vi "Autonomous Independent.vi"   [LabVIEW 2019]
doc: "This VI is called when autonomous begins, and will automatically be terminated when autonomous ends. You can carry out timed or sensor driven robot movement independently without needing to return to the caller."
uses:
  <vilib>/Rock Robotics/WPI/Utilities/WPI_GetSetVariantRefNum.vi
  <vilib>/Rock Robotics/Network Tables/NT Write Numeric Array.vi
  <vilib>/Rock Robotics/Network Tables/NT Read String.vi
panel:
  # "Be sure to right-click and choose Data Operations>>Make Current Value default if you want to save the array values with the VI"
types:
  T1 = typedef "WPI_JoystickDevRef.ctl" = cluster{"Device":T2}
  T2 = typedef "WPI_JoystickDeviceEnum.ctl" = enum16{"USB 0", "USB 1", "USB 2", "USB 3", "USB 4", "USB 5"}
  T3 = typedef "WPI_RobotDriveDevRef.ctl" = cluster{"DevStatus":errorcluster, "Motors[]":T4[], "Square Inputs":bool, "Max Output":dbl}
  T4 = typedef "WPI_MotorControlDeviceRef.ctl" = cluster{"DeviceStatus":errorcluster, "Type":T5, "PWM":cluster{"PWM Channel":T6, "DeadBand":T7}, "CAN":cluster{"Device Number":u8, "SetOutput VI Ref":variant, "GetOutput VI Ref":variant, "Enable VI Ref":variant, "Disable VI Ref":variant, "Data":variant}, "Invert":bool, "DIO PWM":cluster{"PWM \"Enable\" Channel":T6, "DIOChannel":T8, "PWM Rate":dbl}}
  T5 = typedef "WPI_MotorControlType.ctl" = enum16{"PWM", "CAN", "DIO PWM"}
  T6 = typedef "FPGA_DIOPWMChannel.ctl" = enum8{"PWM 0", "PWM 1", "PWM 2", "PWM 3", "PWM 4", "PWM 5", "PWM 6", "PWM 7", "PWM 8", "PWM 9", "PWM MXP 0", "PWM MXP 1", "PWM MXP 2", "PWM MXP 3", "PWM MXP 4", "PWM MXP 5", "PWM MXP 6", "PWM MXP 7", "PWM MXP 8", "PWM MXP 9", "Invalid"}
  T7 = typedef "WPI_PWMDeadband.ctl" = cluster{"Name":string, "maxPositivePwm":i32, "minPositivePwm":i32, "centerPwm":i32, "maxNegativePwm":i32, "minNegativePwm":i32, "angularRange":u16}
  T8 = typedef "FPGA_DIOChannel.ctl" = enum8{"DIO 0", "DIO 1", "DIO 2", "DIO 3", "DIO 4", "DIO 5", "DIO 6", "DIO 7", "DIO 8", "DIO 9", "DIO MXP 0", "DIO MXP 1", "DIO MXP 2", "DIO MXP 3", "DIO MXP 4", "DIO MXP 5", "DIO MXP 6", "DIO MXP 7", "DIO MXP 8", "DIO MXP 9", "DIO MXP 10", "DIO MXP 11", "DIO MXP 12", "DIO MXP 13", "DIO MXP 14", "DIO MXP 15", "SPI Port CS1", "SPI Port CS2", "SPI Port CS3", "SPI Port MISO", "SPI Port MOSI", "Invalid"}
  T9 = typedef "WPI_GyroDevRef.ctl" = cluster{"DevStatus":errorcluster, "Analog Channel":T10, "Gain (VoltsPerDegree/Second)":dbl, "Gyro Type":enum16{"Analog", "XRS450"}, "Handle":i32, "SPI Bus":T11, "Device Found":bool, "Sample Rate":dbl, "Calibrate On Open":bool, "Offset":dbl}
  T10 = typedef "FPGA_AIChannel.ctl" = enum8{"AI 0", "AI 1", "AI 2", "AI 3", "AI MXP 0", "AI MXP 1", "AI MXP 2", "AI MXP 3", "Invalid"}
  T11 = typedef "spi_bus.ctl" = enum16{"SPI On-Board, CS0", "SPI On-Board, CS1", "SPI On-Board, CS2", "SPI On-Board, CS3", "SPI MXP", "Invalid"}
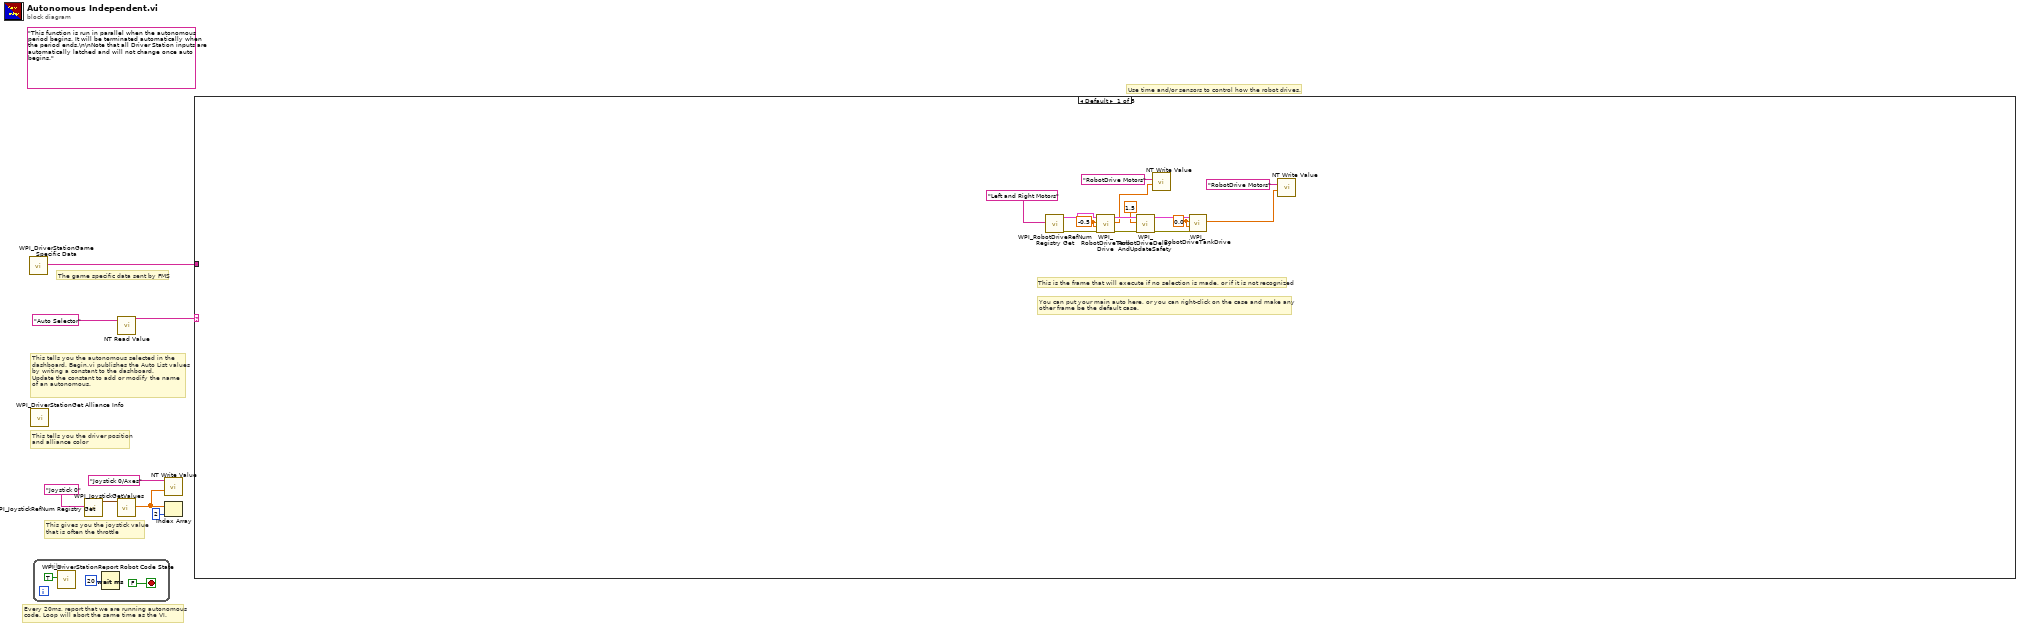
[diagram p0: block diagram]
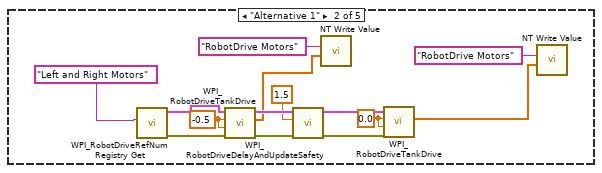
[diagram p2: hidden frame]
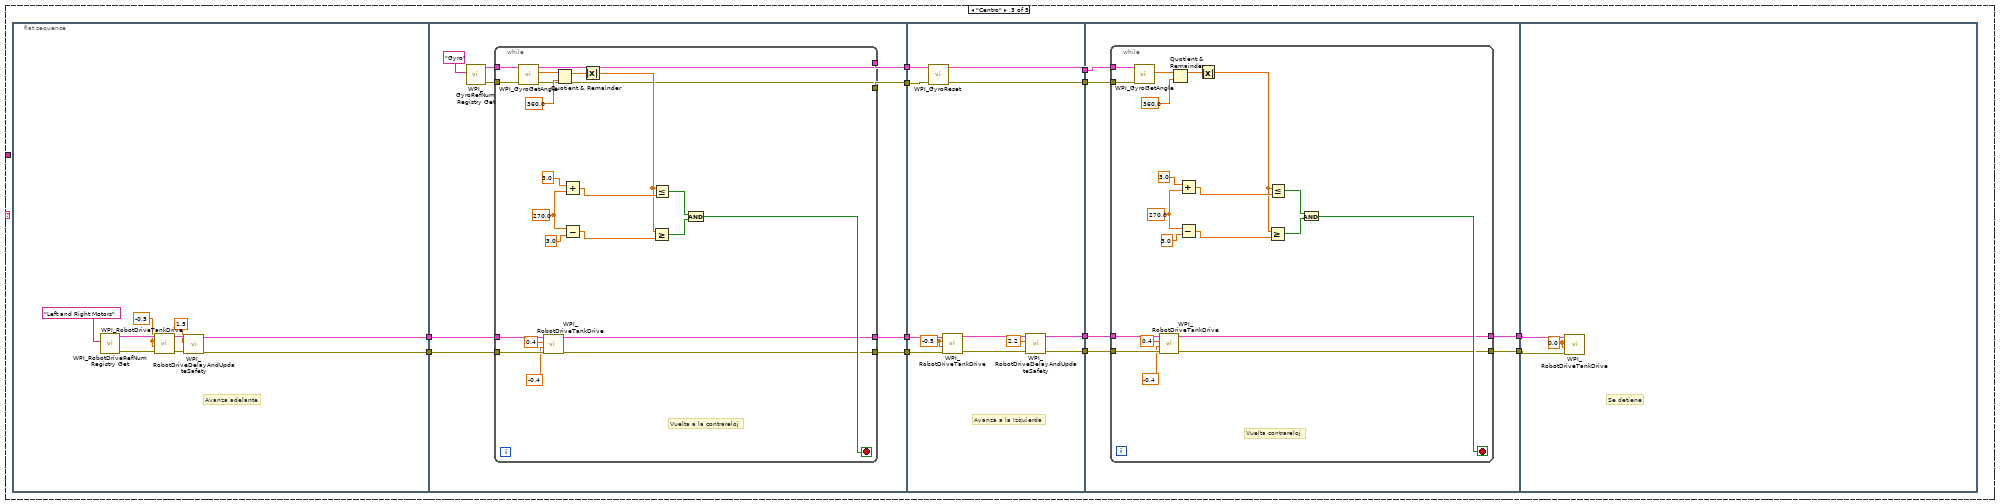
[diagram p3: hidden frame]
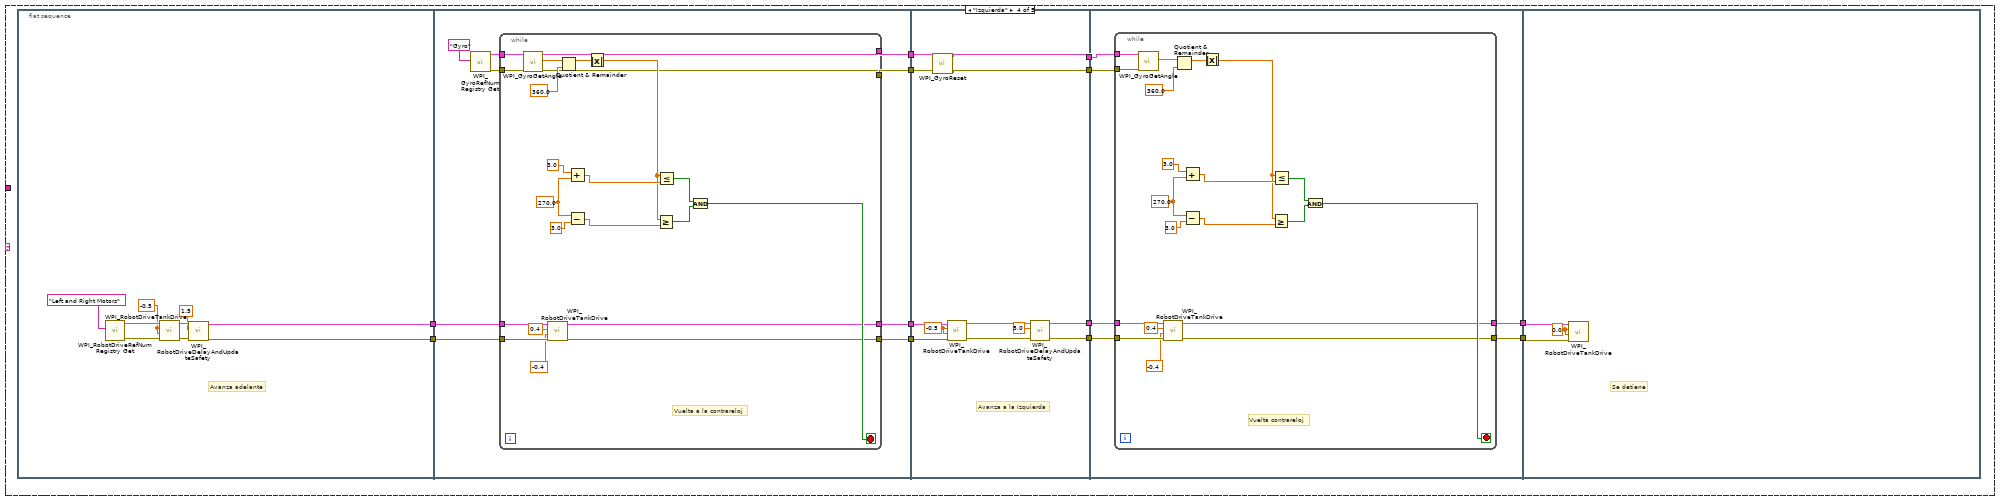
[diagram p4: hidden frame]
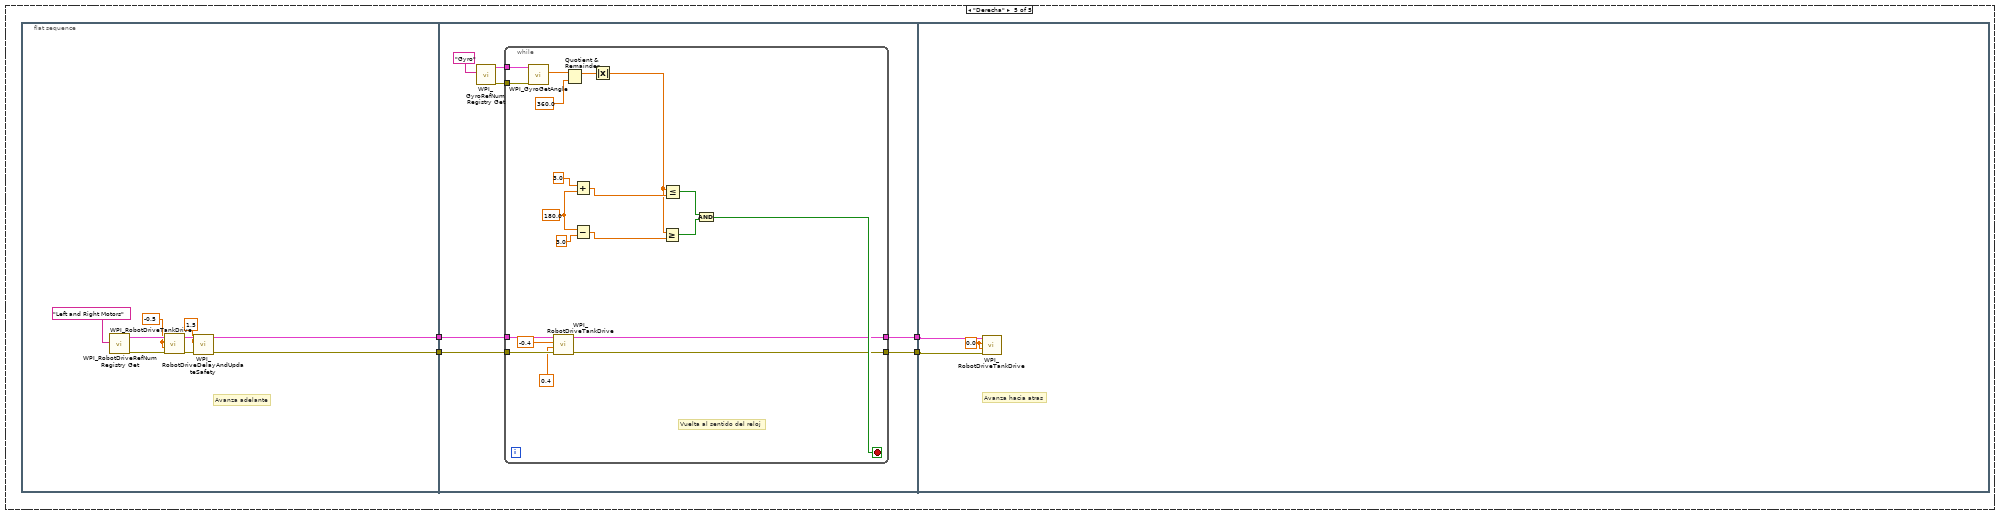
[diagram p5: hidden frame]
diagram:
  (unwired) "This function is run in parallel when the autonomous period begins. It will be terminated automatically when the period ends.\n\nNote that all Driver Station inputs are automatically latched and will not change once auto begins."
  # "The game specific data sent by FMS"
  # "This tells you the autonomous selected in the \ndashboard. Begin.vi publishes the Auto List values\nby writing a constant to the dashboard.\nUpdate the constant to add or modify the name\nof an autonomous."
  # "Every 20ms, report that we are running autonomous\ncode. Loop will abort the same time as the VI."
  # "This gives you the joystick value\nthat is often the throttle"
  # "Use time and/or sensors to control how the robot drives."
  # "This tells you the driver position\nand alliance color"
  n1 = call <vilib>:"WPI_DriverStationGame Specific Data.vi"() -> ("Game Specific Data"=w1:string)  [unwired: 11 in]
  n2 = call <vilib>:"WPI_DriverStationGet Alliance Info.vi"() -> ()  [unwired: 12 out]
  n3 = while {
    stop <- FALSE stop-if-true
    n4 = call <vilib>:"WPI_DriverStationReport Robot Code State.vi"("Autonomous"=TRUE) -> ()  [unwired: 10 in, 1 out]
    n5 = Wait (ms)(milliseconds to wait=u32 20) -> ()  [unwired: 1 out]
  }
  n6 = call <vilib>:"WPI_JoystickRefNum Registry Get.vi"("refnum name"="Joystick 0") -> ("JoystickDevRef"=w7:T1)  [unwired: 1 in, 9 out]
  n7 = call <vilib>:"WPI_JoystickGetValues.vi"("JoystickDevRef"=w7) -> ("Axes"=w3:dbl[])  [unwired: 6 in, 4 out]
  n8 = call-poly <vilib>:"NT Read Value.vi"("Name"="Auto Selector") -> ("String"=w4:string)  [unwired: 9 in, 1 out]
  n9 = call-poly <vilib>:"NT Write Value.vi"("Numeric Array"=w3, "Name"="Joystick 0/Axes") -> ()  [unwired: 9 in, 1 out]
  n10 = Index Array(array=w3, index=2) -> ()  [unwired: 1 out]
  n11 = case shown="Default" w4 {
    tunnel: w1 -> [_ _ _ _ _]
    frame Default {
      w16 = 0.0 ("Left axis value")
      w25 = -0.5 ("Left axis value")
      # "You can put your main auto here, or you can right-click on the case and make any\nother frame be the default case."
      # "This is the frame that will execute if no selection is made, or if it is not recognized"
      n12 = call <vilib>:"WPI_RobotDriveRefNum Registry Get.vi"("refnum name"="Left and Right Motors") -> ("error out"=w23:errorcluster, "RobotDriveDevRef"=w24:T3)  [unwired: 9 in]
      n13 = call <vilib>:"WPI_RobotDriveTankDrive.vi"("error in (no error)"=w23, "Right axis value"=w25, "Left axis value"=w25, "RobotDriveDevRef"=w24) -> ("error out"=w21:errorcluster, "Motor Values"=w13:dbl[], "RobotDriveDevRef"=w22:T3)  [unwired: 5 in]
      n14 = call <vilib>:"WPI_RobotDriveDelayAndUpdateSafety.vi"("error in (no error)"=w21, "Delay (s)"=1.5, "RobotDriveDevRef"=w22) -> ("error out"=w17:errorcluster, "RobotDriveDevRef 2"=w18:T3)  [unwired: 7 in]
      n15 = call-poly <vilib>:"NT Write Value.vi"("Numeric Array"=w13, "Name"="RobotDrive Motors") -> ()  [unwired: 9 in, 1 out]
      n16 = call <vilib>:"WPI_RobotDriveTankDrive.vi"("error in (no error)"=w17, "Right axis value"=w16, "Left axis value"=w16, "RobotDriveDevRef"=w18) -> ("Motor Values"=w12:dbl[])  [unwired: 5 in, 2 out]
      n17 = call-poly <vilib>:"NT Write Value.vi"("Numeric Array"=w12, "Name"="RobotDrive Motors") -> ()  [unwired: 9 in, 1 out]
    }
    frame "Alternative 1" {
      w30 = 0.0 ("Left axis value")
      w39 = -0.5 ("Left axis value")
      n18 = call <vilib>:"WPI_RobotDriveRefNum Registry Get.vi"("refnum name"="Left and Right Motors") -> ("error out"=w37:errorcluster, "RobotDriveDevRef"=w38:T3)  [unwired: 9 in]
      n19 = call <vilib>:"WPI_RobotDriveTankDrive.vi"("error in (no error)"=w37, "Right axis value"=w39, "Left axis value"=w39, "RobotDriveDevRef"=w38) -> ("error out"=w35:errorcluster, "Motor Values"=w27:dbl[], "RobotDriveDevRef"=w36:T3)  [unwired: 5 in]
      n20 = call <vilib>:"WPI_RobotDriveDelayAndUpdateSafety.vi"("error in (no error)"=w35, "Delay (s)"=1.5, "RobotDriveDevRef"=w36) -> ("error out"=w31:errorcluster, "RobotDriveDevRef 2"=w32:T3)  [unwired: 7 in]
      n21 = call-poly <vilib>:"NT Write Value.vi"("Numeric Array"=w27, "Name"="RobotDrive Motors") -> ()  [unwired: 9 in, 1 out]
      n22 = call <vilib>:"WPI_RobotDriveTankDrive.vi"("error in (no error)"=w31, "Right axis value"=w30, "Left axis value"=w30, "RobotDriveDevRef"=w32) -> ("Motor Values"=w26:dbl[])  [unwired: 5 in, 2 out]
      n23 = call-poly <vilib>:"NT Write Value.vi"("Numeric Array"=w26, "Name"="RobotDrive Motors") -> ()  [unwired: 9 in, 1 out]
    }
    frame "Centro" {
      n24 = flat-sequence {
        tunnel: [w53] -> w51
        tunnel: [w52] -> w50
        tunnel: w51 -> [w66]
        tunnel: w50 -> [w65]
        tunnel: [w64] -> w49
        tunnel: [w63] -> w48
        tunnel: [w62] -> w47
        tunnel: [w61] -> w46
        tunnel: w49 -> [w103]
        tunnel: w48 -> [w102]
        tunnel: [w97] -> w45
        tunnel: [w96] -> w44
        tunnel: w47 -> [w95]
        tunnel: w46 -> [w94]
        tunnel: [w93] -> w43
        tunnel: [w92] -> w42
        tunnel: w45 -> [w109]
        tunnel: w44 -> [w108]
        tunnel: w43 -> [w107]
        tunnel: w42 -> [w106]
        tunnel: [w105] -> w41
        tunnel: [w104] -> w40
        tunnel: w41 -> [w131]
        tunnel: w40 -> [w130]
        frame #0 {
          w57 = -0.5 ("Right axis value")
          # "Avanza adelante"
          n25 = call <vilib>:"WPI_RobotDriveRefNum Registry Get.vi"("refnum name"="Left and Right Motors") -> ("error out"=w59:errorcluster, "RobotDriveDevRef"=w58:T3)  [unwired: 9 in]
          n26 = call <vilib>:"WPI_RobotDriveTankDrive.vi"("error in (no error)"=w59, "Right axis value"=w57, "Left axis value"=w57, "RobotDriveDevRef"=w58) -> ("error out"=w56:errorcluster, "RobotDriveDevRef"=w55:T3)  [unwired: 5 in, 1 out]
          n27 = call <vilib>:"WPI_RobotDriveDelayAndUpdateSafety.vi"("error in (no error)"=w56, "Delay (s)"=1.5, "RobotDriveDevRef"=w55) -> ("error out"=w52:errorcluster, "RobotDriveDevRef 2"=w53:T3)  [unwired: 7 in]
        }
        frame #1 {
          n28 = call <vilib>:"WPI_GyroRefNum Registry Get.vi"("refnum name"="Gyro") -> ("error out"=w68:errorcluster, "GyroDevRef"=w67:T9)  [unwired: 9 in]
          n29 = while {
            tunnel: w68 -> [w88]
            tunnel: w67 -> [w87]
            tunnel: w66 -> [w85]
            tunnel: w65 -> [w86]
            tunnel: [w73] -> w64
            tunnel: [w72] -> w63
            tunnel: [w71] -> w62
            tunnel: [w70] -> w61
            stop <- w74 stop-if-true
            w81 = 270.0 ("y")
            # "Vuelta a la contrareloj"
            n30 = call <vilib>:"WPI_GyroGetAngle.vi"("error in"=w88, "GyroDevRef"=w87) -> ("error out"=w70:errorcluster, "Angle"=w91:dbl, "GyroDevRef"=w71:T9)  [unwired: 5 in, 2 out]
            n31 = call <vilib>:"WPI_RobotDriveTankDrive.vi"("error in (no error)"=w86, "Right axis value"=-0.4, "Left axis value"=0.4, "RobotDriveDevRef"=w85) -> ("error out"=w72:errorcluster, "RobotDriveDevRef"=w73:T3)  [unwired: 5 in, 1 out]
            n32 = Quotient & Remainder(x=w91, y=360.0) -> (x-y*floor(x/y)=w89:dbl)  [unwired: 1 out]
            n33 = Add(x=3.0, y=w81) -> (x+y=w79:dbl)
            n34 = Subtract(x=w81, y=3.0) -> (x-y=w78:dbl)
            n35 = Absolute Value(x=w89) -> (abs(x)=w75:dbl)
            n36 = Greater Or Equal?(x=w75, y=w78) -> (x >= y?=w76:bool)
            n37 = Less Or Equal?(x=w75, y=w79) -> (x <= y?=w77:bool)
            n38 = And(x=w77, y=w76) -> (x .and. y?=w74:bool)
          }
        }
        frame #2 {
          w101 = -0.5 ("Left axis value")
          # "Avanza a la Izquierda"
          n39 = call <vilib>:"WPI_GyroReset.vi"("error in"=w94, "GyroDevRef"=w95) -> ("error out"=w92:errorcluster, "GyroDevRef"=w93:T9)  [unwired: 8 in]
          n40 = call <vilib>:"WPI_RobotDriveTankDrive.vi"("error in (no error)"=w102, "Right axis value"=w101, "Left axis value"=w101, "RobotDriveDevRef"=w103) -> ("error out"=w99:errorcluster, "RobotDriveDevRef"=w100:T3)  [unwired: 5 in, 1 out]
          n41 = call <vilib>:"WPI_RobotDriveDelayAndUpdateSafety.vi"("error in (no error)"=w99, "Delay (s)"=2.2, "RobotDriveDevRef"=w100) -> ("error out"=w96:errorcluster, "RobotDriveDevRef 2"=w97:T3)  [unwired: 7 in]
        }
        frame #3 {
          n42 = while {
            tunnel: w106 -> [w126]
            tunnel: w107 -> [w125]
            tunnel: w109 -> [w123]
            tunnel: w108 -> [w124]
            tunnel: [w111] -> w105
            tunnel: [w110] -> w104
            stop <- w112 stop-if-true
            w119 = 270.0 ("y")
            # "Vuelta contrareloj"
            n43 = call <vilib>:"WPI_GyroGetAngle.vi"("error in"=w126, "GyroDevRef"=w125) -> ("Angle"=w129:dbl)  [unwired: 5 in, 4 out]
            n44 = call <vilib>:"WPI_RobotDriveTankDrive.vi"("error in (no error)"=w124, "Right axis value"=-0.4, "Left axis value"=0.4, "RobotDriveDevRef"=w123) -> ("error out"=w110:errorcluster, "RobotDriveDevRef"=w111:T3)  [unwired: 5 in, 1 out]
            n45 = Quotient & Remainder(x=w129, y=360.0) -> (x-y*floor(x/y)=w127:dbl)  [unwired: 1 out]
            n46 = Add(x=3.0, y=w119) -> (x+y=w117:dbl)
            n47 = Subtract(x=w119, y=3.0) -> (x-y=w116:dbl)
            n48 = Absolute Value(x=w127) -> (abs(x)=w113:dbl)
            n49 = Greater Or Equal?(x=w113, y=w116) -> (x >= y?=w114:bool)
            n50 = Less Or Equal?(x=w113, y=w117) -> (x <= y?=w115:bool)
            n51 = And(x=w115, y=w114) -> (x .and. y?=w112:bool)
          }
        }
        frame #4 {
          w132 = 0.0 ("Left axis value")
          # "Se detiene"
          n52 = call <vilib>:"WPI_RobotDriveTankDrive.vi"("error in (no error)"=w130, "Right axis value"=w132, "Left axis value"=w132, "RobotDriveDevRef"=w131) -> ()  [unwired: 5 in, 3 out]
        }
      }
    }
    frame "Izquierda" {
      n53 = flat-sequence {
        tunnel: [w146] -> w144
        tunnel: [w145] -> w143
        tunnel: w144 -> [w159]
        tunnel: w143 -> [w158]
        tunnel: [w157] -> w142
        tunnel: [w156] -> w141
        tunnel: [w155] -> w140
        tunnel: [w154] -> w139
        tunnel: w142 -> [w196]
        tunnel: w141 -> [w195]
        tunnel: [w190] -> w138
        tunnel: [w189] -> w137
        tunnel: w140 -> [w188]
        tunnel: w139 -> [w187]
        tunnel: [w186] -> w136
        tunnel: [w185] -> w135
        tunnel: w138 -> [w202]
        tunnel: w137 -> [w201]
        tunnel: w136 -> [w200]
        tunnel: w135 -> [w199]
        tunnel: [w198] -> w134
        tunnel: [w197] -> w133
        tunnel: w134 -> [w224]
        tunnel: w133 -> [w223]
        frame #0 {
          w150 = -0.5 ("Right axis value")
          # "Avanza adelante"
          n54 = call <vilib>:"WPI_RobotDriveRefNum Registry Get.vi"("refnum name"="Left and Right Motors") -> ("error out"=w152:errorcluster, "RobotDriveDevRef"=w151:T3)  [unwired: 9 in]
          n55 = call <vilib>:"WPI_RobotDriveTankDrive.vi"("error in (no error)"=w152, "Right axis value"=w150, "Left axis value"=w150, "RobotDriveDevRef"=w151) -> ("error out"=w149:errorcluster, "RobotDriveDevRef"=w148:T3)  [unwired: 5 in, 1 out]
          n56 = call <vilib>:"WPI_RobotDriveDelayAndUpdateSafety.vi"("error in (no error)"=w149, "Delay (s)"=1.5, "RobotDriveDevRef"=w148) -> ("error out"=w145:errorcluster, "RobotDriveDevRef 2"=w146:T3)  [unwired: 7 in]
        }
        frame #1 {
          n57 = call <vilib>:"WPI_GyroRefNum Registry Get.vi"("refnum name"="Gyro") -> ("error out"=w161:errorcluster, "GyroDevRef"=w160:T9)  [unwired: 9 in]
          n58 = while {
            tunnel: w161 -> [w181]
            tunnel: w160 -> [w180]
            tunnel: w159 -> [w178]
            tunnel: w158 -> [w179]
            tunnel: [w166] -> w157
            tunnel: [w165] -> w156
            tunnel: [w164] -> w155
            tunnel: [w163] -> w154
            stop <- w167 stop-if-true
            w174 = 270.0 ("y")
            # "Vuelta a la contrareloj"
            n59 = call <vilib>:"WPI_GyroGetAngle.vi"("error in"=w181, "GyroDevRef"=w180) -> ("error out"=w163:errorcluster, "Angle"=w184:dbl, "GyroDevRef"=w164:T9)  [unwired: 5 in, 2 out]
            n60 = call <vilib>:"WPI_RobotDriveTankDrive.vi"("error in (no error)"=w179, "Right axis value"=-0.4, "Left axis value"=0.4, "RobotDriveDevRef"=w178) -> ("error out"=w165:errorcluster, "RobotDriveDevRef"=w166:T3)  [unwired: 5 in, 1 out]
            n61 = Quotient & Remainder(x=w184, y=360.0) -> (x-y*floor(x/y)=w182:dbl)  [unwired: 1 out]
            n62 = Add(x=3.0, y=w174) -> (x+y=w172:dbl)
            n63 = Subtract(x=w174, y=3.0) -> (x-y=w171:dbl)
            n64 = Absolute Value(x=w182) -> (abs(x)=w168:dbl)
            n65 = Greater Or Equal?(x=w168, y=w171) -> (x >= y?=w169:bool)
            n66 = Less Or Equal?(x=w168, y=w172) -> (x <= y?=w170:bool)
            n67 = And(x=w170, y=w169) -> (x .and. y?=w167:bool)
          }
        }
        frame #2 {
          w194 = -0.5 ("Left axis value")
          # "Avanza a la Izquierda"
          n68 = call <vilib>:"WPI_GyroReset.vi"("error in"=w187, "GyroDevRef"=w188) -> ("error out"=w185:errorcluster, "GyroDevRef"=w186:T9)  [unwired: 8 in]
          n69 = call <vilib>:"WPI_RobotDriveTankDrive.vi"("error in (no error)"=w195, "Right axis value"=w194, "Left axis value"=w194, "RobotDriveDevRef"=w196) -> ("error out"=w192:errorcluster, "RobotDriveDevRef"=w193:T3)  [unwired: 5 in, 1 out]
          n70 = call <vilib>:"WPI_RobotDriveDelayAndUpdateSafety.vi"("error in (no error)"=w192, "Delay (s)"=5.0, "RobotDriveDevRef"=w193) -> ("error out"=w189:errorcluster, "RobotDriveDevRef 2"=w190:T3)  [unwired: 7 in]
        }
        frame #3 {
          n71 = while {
            tunnel: w199 -> [w219]
            tunnel: w200 -> [w218]
            tunnel: w202 -> [w216]
            tunnel: w201 -> [w217]
            tunnel: [w204] -> w198
            tunnel: [w203] -> w197
            stop <- w205 stop-if-true
            w212 = 270.0 ("y")
            # "Vuelta contrareloj"
            n72 = call <vilib>:"WPI_GyroGetAngle.vi"("error in"=w219, "GyroDevRef"=w218) -> ("Angle"=w222:dbl)  [unwired: 5 in, 4 out]
            n73 = call <vilib>:"WPI_RobotDriveTankDrive.vi"("error in (no error)"=w217, "Right axis value"=-0.4, "Left axis value"=0.4, "RobotDriveDevRef"=w216) -> ("error out"=w203:errorcluster, "RobotDriveDevRef"=w204:T3)  [unwired: 5 in, 1 out]
            n74 = Quotient & Remainder(x=w222, y=360.0) -> (x-y*floor(x/y)=w220:dbl)  [unwired: 1 out]
            n75 = Add(x=3.0, y=w212) -> (x+y=w210:dbl)
            n76 = Subtract(x=w212, y=3.0) -> (x-y=w209:dbl)
            n77 = Absolute Value(x=w220) -> (abs(x)=w206:dbl)
            n78 = Greater Or Equal?(x=w206, y=w209) -> (x >= y?=w207:bool)
            n79 = Less Or Equal?(x=w206, y=w210) -> (x <= y?=w208:bool)
            n80 = And(x=w208, y=w207) -> (x .and. y?=w205:bool)
          }
        }
        frame #4 {
          w225 = 0.0 ("Left axis value")
          # "Se detiene"
          n81 = call <vilib>:"WPI_RobotDriveTankDrive.vi"("error in (no error)"=w223, "Right axis value"=w225, "Left axis value"=w225, "RobotDriveDevRef"=w224) -> ()  [unwired: 5 in, 3 out]
        }
      }
    }
    frame "Derecha" {
      n82 = flat-sequence {
        tunnel: [w231] -> w229
        tunnel: [w230] -> w228
        tunnel: w229 -> [w242]
        tunnel: w228 -> [w241]
        tunnel: [w240] -> w227
        tunnel: [w239] -> w226
        tunnel: w227 -> [w267]
        tunnel: w226 -> [w266]
        frame #0 {
          w235 = -0.5 ("Right axis value")
          # "Avanza adelante"
          n83 = call <vilib>:"WPI_RobotDriveRefNum Registry Get.vi"("refnum name"="Left and Right Motors") -> ("error out"=w237:errorcluster, "RobotDriveDevRef"=w236:T3)  [unwired: 9 in]
          n84 = call <vilib>:"WPI_RobotDriveTankDrive.vi"("error in (no error)"=w237, "Right axis value"=w235, "Left axis value"=w235, "RobotDriveDevRef"=w236) -> ("error out"=w234:errorcluster, "RobotDriveDevRef"=w233:T3)  [unwired: 5 in, 1 out]
          n85 = call <vilib>:"WPI_RobotDriveDelayAndUpdateSafety.vi"("error in (no error)"=w234, "Delay (s)"=1.5, "RobotDriveDevRef"=w233) -> ("error out"=w230:errorcluster, "RobotDriveDevRef 2"=w231:T3)  [unwired: 7 in]
        }
        frame #1 {
          n86 = call <vilib>:"WPI_GyroRefNum Registry Get.vi"("refnum name"="Gyro") -> ("error out"=w244:errorcluster, "GyroDevRef"=w243:T9)  [unwired: 9 in]
          n87 = while {
            tunnel: w244 -> [w262]
            tunnel: w243 -> [w261]
            tunnel: w242 -> [w259]
            tunnel: w241 -> [w260]
            tunnel: [w247] -> w240
            tunnel: [w246] -> w239
            stop <- w248 stop-if-true
            w255 = 180.0 ("y")
            # "Vuelta al sentido del reloj"
            n88 = call <vilib>:"WPI_GyroGetAngle.vi"("error in"=w262, "GyroDevRef"=w261) -> ("Angle"=w265:dbl)  [unwired: 5 in, 4 out]
            n89 = call <vilib>:"WPI_RobotDriveTankDrive.vi"("error in (no error)"=w260, "Right axis value"=0.4, "Left axis value"=-0.4, "RobotDriveDevRef"=w259) -> ("error out"=w246:errorcluster, "RobotDriveDevRef"=w247:T3)  [unwired: 5 in, 1 out]
            n90 = Quotient & Remainder(x=w265, y=360.0) -> (x-y*floor(x/y)=w263:dbl)  [unwired: 1 out]
            n91 = Add(x=3.0, y=w255) -> (x+y=w253:dbl)
            n92 = Subtract(x=w255, y=3.0) -> (x-y=w252:dbl)
            n93 = Absolute Value(x=w263) -> (abs(x)=w249:dbl)
            n94 = Greater Or Equal?(x=w249, y=w252) -> (x >= y?=w250:bool)
            n95 = Less Or Equal?(x=w249, y=w253) -> (x <= y?=w251:bool)
            n96 = And(x=w251, y=w250) -> (x .and. y?=w248:bool)
          }
        }
        frame #2 {
          w268 = 0.0 ("Left axis value")
          # "Avanza hacia atras"
          n97 = call <vilib>:"WPI_RobotDriveTankDrive.vi"("error in (no error)"=w266, "Right axis value"=w268, "Left axis value"=w268, "RobotDriveDevRef"=w267) -> ()  [unwired: 5 in, 3 out]
        }
      }
    }
  }
